vi "Remote Calibration Panel.vi"() -> ()   [LabVIEW 2014]
uses:
  Formula Hybrid 2012 r1/Remote Calibration/Remote Calibration Typedef.ctl
panel:
  in  "Send Cal to Car":bool
  in  "Cal":T1={"Rear BP Scaling Factor"=1250.0, "Front BP Scaling Factor"=1250.0, "Rear BP Offset (V)"=0.4820899963378906, "Front BP Offset"=0.4808177947998047, "Throttle 2 Max"=0.27001953125, "Throttle 2 Min"=0.489990234375, "Throttle 1 Max"=0.6201171875, "Throttle 1 Min"=0.41015625, "MC Update Period (ms)"=200, "Regen Mult."=0.0, "Zero Torque %"=0.0, "Torque Mult."=160.0, "Activation Brake Pressure"=-1.0}
  in  "Load Cal From Car":bool
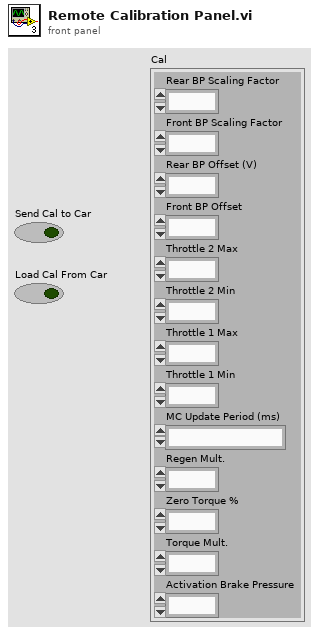
[diagram p1: front panel]
types:
  T1 = typedef "Remote Calibration Typedef.ctl" = cluster{"Rear BP Scaling Factor":fxp<+,11,11>, "Front BP Scaling Factor":fxp<+,11,11>, "Rear BP Offset (V)":fxp<+/-,26,5>, "Front BP Offset":fxp<+/-,26,5>, "Throttle 2 Max":fxp<+,16,4>, "Throttle 2 Min":fxp<+,16,4>, "Throttle 1 Max":fxp<+,16,4>, "Throttle 1 Min":fxp<+,16,4>, "MC Update Period (ms)":u32, "Regen Mult.":dbl, "Zero Torque %":dbl, "Torque Mult.":dbl, "Activation Brake Pressure":dbl}
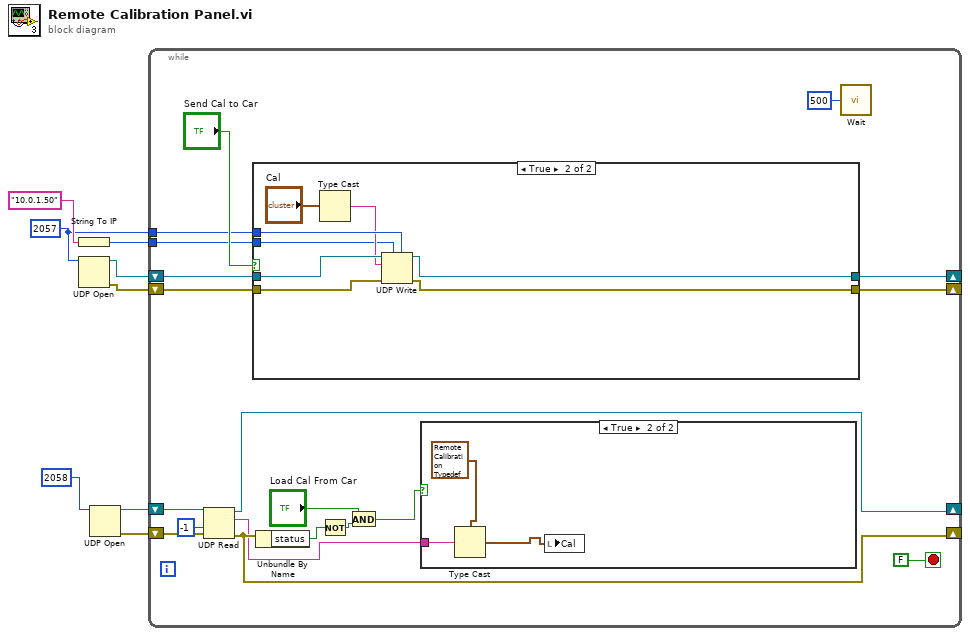
[diagram p0: block diagram]
diagram:
  w2 = u16 2057 ("port")
  n1 = String To IP(1:"10.0.1.50" ("name")) -> (0:w1:u32)
  n2 = UDP Open(11:w2) -> (port=w4:refnum<k16>, 0:w3:errorcluster)  [unwired: 4 in, 1 out]
  n3 = UDP Open(11:u16 2058 ("port")) -> (port=w7:refnum<k16>, 0:w6:errorcluster)  [unwired: 4 in, 1 out]
  n4 = while {
    shift-right: [w21] -> _
    shift-left: w7 -> [w26]
    shift-right: [w20] -> _
    shift-left: w6 -> [w25]
    tunnel: w2 -> [w15]
    shift-right: [w14] -> _
    shift-left: w4 -> [w17]
    shift-right: [w13] -> _
    shift-left: w3 -> [w16]
    tunnel: w1 -> [w12]
    stop <- FALSE stop-if-true
    n5 = UDP Read(connection ID=w26, timeout ms (25000)=-1, 8:w25) -> (data out=w19:string, error out=w20:errorcluster, 3:w21:refnum<k16>)  [unwired: 1 in, 2 out]
    n6 = case shown="True" "Send Cal to Car" {
      tunnel: w17 -> [w29 w37]
      tunnel: w16 -> [w28 w36]
      tunnel: w15 -> [_ w35]
      tunnel: [w29 w33] -> w14
      tunnel: [w28 w32] -> w13
      tunnel: w12 -> [_ w31]
      frame False {
      }
      frame True {
        n7 = Type Cast(x="Cal") -> (*(type *) &x=w34:string)  [unwired: 1 in]
        n8 = UDP Write(address=w31, port or service name=w35, connection ID=w37, data in=w34, 8:w36) -> (error out=w32:errorcluster, 3:w33:refnum<k16>)  [unwired: 1 in]
      }
    }
    n9 = Unbundle By Name(w20) -> ("status"=w9:bool)
    n10 = Not(x=w9) -> (.not. x?=w10:bool)
    n11 = And(x="Load Cal From Car", y=w10) -> (x .and. y?=w23:bool)
    n12 = case shown="True" w23 {
      tunnel: w19 -> [_ w40]
      frame False {
      }
      frame True {
        n13 = Type Cast(type=T1 {"Rear BP Scaling Factor"=1250.0, "Front BP Scaling Factor"=1250.0, "Rear BP Offset (V)"=0.4820899963378906, "Front BP Offset"=0.4808177947998047, "Throttle 2 Max"=3.89990234375, "Throttle 2 Min"=2.090087890625, "Throttle 1 Max"=0.6298828125, "Throttle 1 Min"=2.4599609375, "MC Update Period (ms)"=20, "Regen Mult."=0.0, "Zero Torque %"=0.0, "Torque Mult."=160.0, "Activation Brake Pressure"=50.0} ("Remote Calibration Parameters"), x=w40) -> (*(type *) &x=w38:T1)
        n14 = local write "Cal"(w38) -> ()
      }
    }
    n15 = call "Wait"("Count(mSec)"=u32 500) -> ()  [unwired: 1 out]
  }
